vi "CTRE_Phoenix_CANcoder_ConfigSensorDirection.vi"(6 "timeoutMs":i32, 8 "error in":errorcluster, 10 "Sensor Direction":bool=TRUE, 11 "CTRE_CANcoder_DeviceRef":T1) -> (0 "error out":errorcluster, 3 "CTRE_CANcoder_DeviceRef":T1)   [LabVIEW 2019]
doc: "Choose which direction is interpreted as positive displacement. This affects both \"Position\" and \"Absolute Position\".\n\n<b>Sensor Direction</b> False (default) means positive rotation occurs when magnet is spun counter-clockwise when observer is facing the LED side of CANCoder.\n<b>timeoutMs</b> Timeout value in ms. If nonzero, function will wait for config success and report an error if it times out. If zero, no blocking or checking is performed."
uses:
  <vilib>/Rock Robotics/WPI/ThirdParty/Phoenix-LabVIEW/CANCoder/Controls/CTRE_Phoenix_CANcoder_DeviceRef.ctl
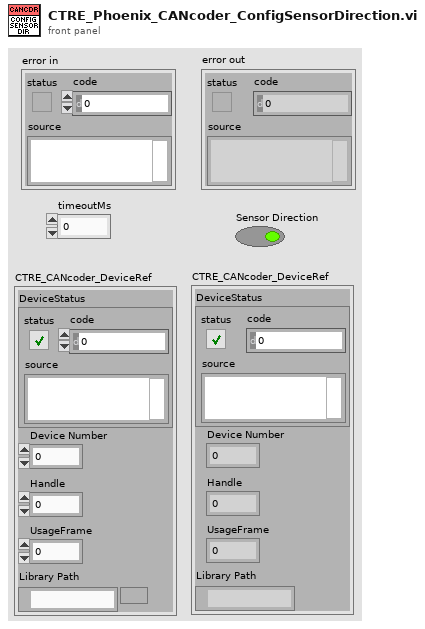
[diagram p1: front panel]
types:
  T1 = typedef "CTRE_Phoenix_CANcoder_DeviceRef.ctl" = cluster{"DeviceStatus":errorcluster, "Device Number":u8, "Handle":u64, "UsageFrame":u32, "Library Path":path}
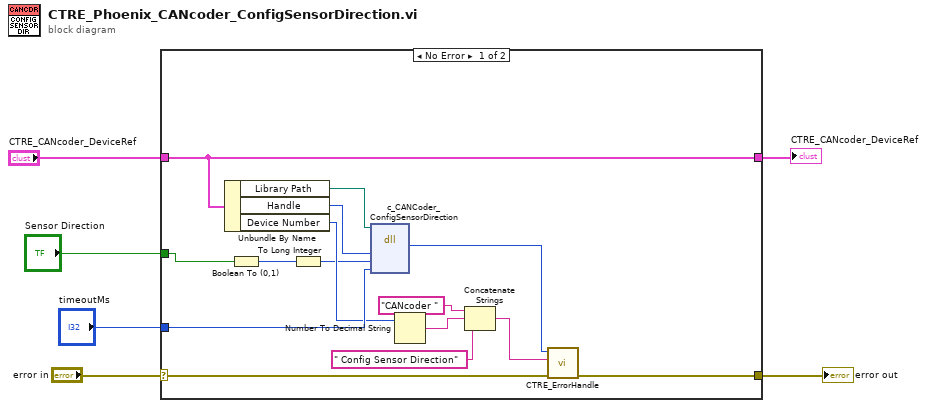
[diagram p0: block diagram]
diagram:
  n1 = case shown="No Error" "error in" {
    selector: "error in" -> [w18 w23]
    tunnel: "CTRE_CANcoder_DeviceRef" -> [w19 w22]
    tunnel: [w17 w23] -> w5
    tunnel: [w19 w22] -> w2
    tunnel: "timeoutMs" -> [w15 _]
    tunnel: "Sensor Direction" -> [w9 _]
    frame No Error {
      n2 = Unbundle By Name(w19) -> ("Library Path"=w21:path, "Handle"=w20:u64, "Device Number"=w10:u8)
      n3 = Boolean To (0,1)(Boolean=w9) -> (0, 1=w8:i16)
      n4 = To Long Integer(number=w8) -> (32bit integer=w7:i32)
      n5 = dll-call lib="?" fn="c_CANCoder_ConfigSensorDirection"(path in=w21, "handle"=w20, "bDirection"=w7, "timeoutMs"=w15) -> ("CTR_Code"=w16:i8)  [unwired: 5 in, 2 out]
      n6 = Number To Decimal String(number=w10) -> (decimal integer string=w14:string)  [unwired: 1 in]
      n7 = Concatenate Strings("CANcoder " ("string"), w14, " Config Sensor Direction" ("string")) -> (w11:string)
      n8 = call <vilib>:"CTRE_ErrorHandle.vi"("error in"=w18, "origin"=w11, "code"=w16) -> ("error out"=w17:errorcluster)  [unwired: 8 in]
    }
    frame Error {
    }
  }
  "error out" <- w5
  "CTRE_CANcoder_DeviceRef" <- w2
